vi "Noise.Buffer.vi"(2 "Action":T1(ring), 5 "Npts":i32, 7 "Data In":dbl[](array[numeric]), 9 "Name":string, 11 "error in (no error)":errorcluster, 12 "offset":i32=-1) -> (8 "Data Out":dbl[](array[numeric]), 15 "error out":errorcluster)   [LabVIEW 2020]
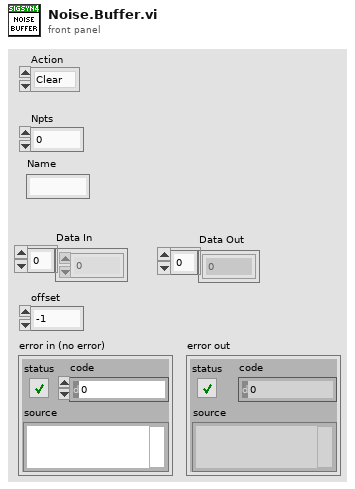
[diagram p1: front panel]
types:
  T1 = enum16{"Clear", "Set data", "Reset index", "Get data"}
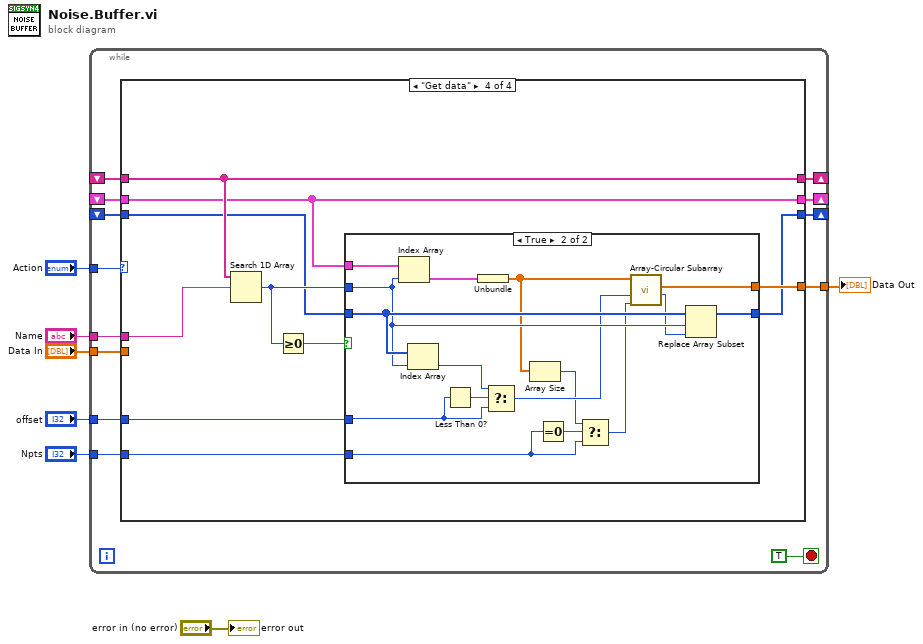
[diagram p0: block diagram]
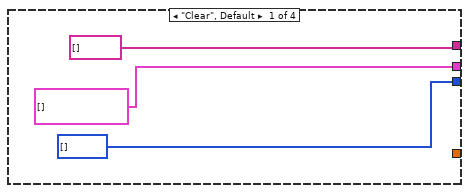
[diagram p2: hidden frame]
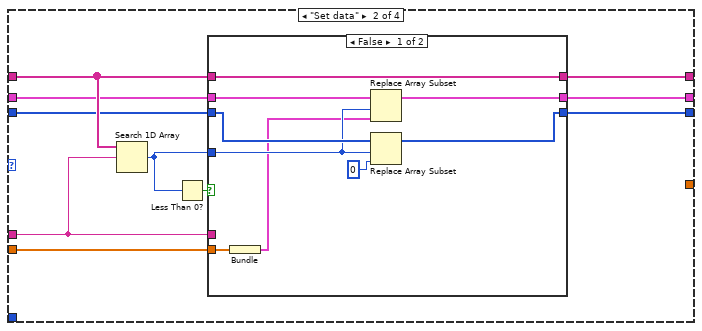
[diagram p3: hidden frame]
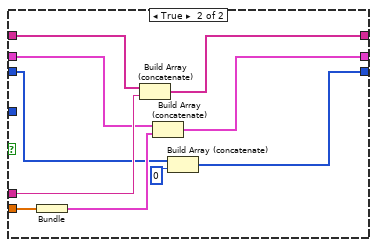
[diagram p4: hidden frame]
diagram:
  n1 = while {
    shift-right: [w19] -> _
    shift-left: _ -> [w18]
    shift-right: [w17] -> _
    shift-left: _ -> [w16]
    tunnel: "Action" -> [w15]
    shift-right: [w14] -> _
    shift-left: _ -> [w13]
    tunnel: "Name" -> [w12]
    tunnel: "Data In" -> [w11]
    tunnel: "Npts" -> [w10]
    tunnel: [w9] -> w3
    tunnel: "offset" -> [w8]
    stop <- TRUE stop-if-true
    n2 = case shown="\"Get data\"" w15 {
      tunnel: [string[] [] w27 w55 w64] -> w19
      tunnel: w18 -> [_ w32 w55 w64]
      tunnel: [cluster{dbl[]}[] [] w26 w54 w62] -> w17
      tunnel: w16 -> [_ w31 w54 w62]
      tunnel: [i32[] [] w25 w53 w57] -> w14
      tunnel: w13 -> [_ w30 w53 w59]
      tunnel: w12 -> [_ w28 _ w65]
      tunnel: w11 -> [_ w29 _ _]
      tunnel: w10 -> [_ _ _ w60]
      tunnel: [_ _ _ w58] -> w9
      tunnel: w8 -> [_ _ _ w56]
      frame "Clear", Default {
      }
      frame "Set data" {
        n3 = Search 1D Array(1D array=w32, element=w28) -> (index of element=w24:i32)  [unwired: 1 in]
        n4 = Less Than 0?(x=w24) -> (x < 0?=w33:bool)
        n5 = case shown="False" w33 {
          tunnel: w32 -> [w42 w52]
          tunnel: w31 -> [w38 w47]
          tunnel: w30 -> [w41 w45]
          tunnel: w29 -> [w35 w49]
          tunnel: w28 -> [_ w51]
          tunnel: [w42 w50] -> w27
          tunnel: [w37 w46] -> w26
          tunnel: [w39 w43] -> w25
          tunnel: w24 -> [w36 _]
          frame False {
            n6 = Bundle("Data In"=w35) -> (w34:cluster{"Data In":dbl[]})  [unwired: 1 in]
            n7 = Replace Array Subset(array=w38, new element=w34, index=w36) -> (w37:cluster{"Data In":dbl[]}[])
            n8 = Replace Array Subset(array=w41, new element=0 ("new element/subarray"), index=w36) -> (w39:i32[])
          }
          frame True {
            n9 = Bundle("Data In"=w49) -> (w48:cluster{"Data In":dbl[]})  [unwired: 1 in]
            n10 = Build Array (concatenate)(w52, w51) -> (w50:string[])
            n11 = Build Array (concatenate)(w47, w48) -> (w46:cluster{"Data In":dbl[]}[])
            n12 = Build Array (concatenate)(w45, 0) -> (w43:i32[])
          }
        }
      }
      frame "Reset index" {
      }
      frame "Get data" {
        n13 = Search 1D Array(1D array=w64, element=w65) -> (index of element=w61:i32)  [unwired: 1 in]
        n14 = Greater Or Equal To 0?(x=w61) -> (x >= 0?=w63:bool)
        n15 = case shown="True" w63 {
          tunnel: w62 -> [_ w82]
          tunnel: w61 -> [_ w78]
          tunnel: w60 -> [_ w70]
          tunnel: w59 -> [w66 w79]
          tunnel: [_ w80] -> w58
          tunnel: [w66 w76] -> w57
          tunnel: w56 -> [_ w72]
          frame False {
          }
          frame True {
            n16 = Index Array(array=w82, index=w78) -> (element=w81:cluster{"Data In":dbl[]})
            n17 = Index Array(array=w79, index=w78) -> (element=w75:i32)
            n18 = Less Than 0?(x=w72) -> (x < 0?=w73:bool)
            n19 = Unbundle(w81) -> ("Data In"=w68:dbl[])
            n20 = Select(t=w75, s=w73, f=w72) -> (s? t:f=w74:i32)
            n21 = Array Size(array=w68) -> (size(s)=w67:i32)
            n22 = Equal To 0?(x=w70) -> (x = 0?=w71:bool)
            n23 = Select(t=w67, s=w71, f=w70) -> (s? t:f=w69:i32)
            n24 = call "Array-Circular Subarray.vi"("Npts"=w69, "Offset (in)"=w74, "Array"=w68) -> ("Offset (out)"=w77:i32, "Subarray"=w80:dbl[])  [unwired: 7 in]
            n25 = Replace Array Subset(array=w79, new element=w77, index=w78) -> (w76:i32[])
          }
        }
      }
    }
  }
  "Data Out" <- w3
  "error out" <- "error in (no error)"
